vi "get_terminals.vi"(0 "ClockDL100201DAQmx in":refnum<class "ClockMT120808DAQmxSimple.lvclass">, 11 "error in (no error)":errorcluster) -> (4 "ClockDL100201DAQmx out":refnum<class "ClockMT120808DAQmxSimple.lvclass">, 6 "counter":tag, 15 "error out":errorcluster)   [LabVIEW 2010, in "ClockMT120808DAQmxSimple.lvclass"]
uses:
  ClockMT120808DAQmxSimple.lvclass
  ClockMT120808DAQmxSimple.lvclass/ClockMT120808DAQmxSimple.ctl
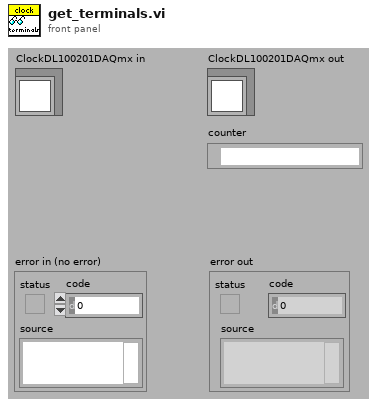
[diagram p1: front panel]
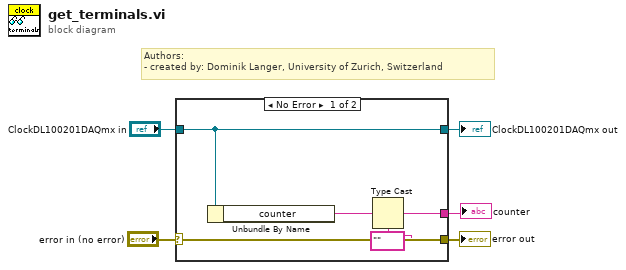
[diagram p0: block diagram]
diagram:
  # "Authors: \n- created by: Dominik Langer, University of Zurich, Switzerland"
  n1 = case shown="No Error" "error in (no error)" {
    selector: "error in (no error)" -> [w10 w12]
    tunnel: [w10 w12] -> w4
    tunnel: [w9 w11] -> w2
    tunnel: "ClockDL100201DAQmx in" -> [w9 w11]
    tunnel: [w7 _] -> w1
    frame No Error {
      n2 = Unbundle By Name(w9) -> ("counter"=w8:string)
      n3 = Type Cast(type=tag "" ("counter"), x=w8) -> (*(type *) &x=w7:tag)
    }
    frame Error {
    }
  }
  "error out" <- w4
  "ClockDL100201DAQmx out" <- w2
  "counter" <- w1
